vi "Write to Dashboard.vi"   [LabVIEW 2014]
uses:
  Global Variables/Sensor Data (Edited).vi
  <vilib>/Rock Robotics/Network Tables/SD Write Number.vi
  <vilib>/Rock Robotics/Network Tables/SD Write Numeric Array.vi
  <vilib>/Rock Robotics/Network Tables/SD Write Boolean Array.vi
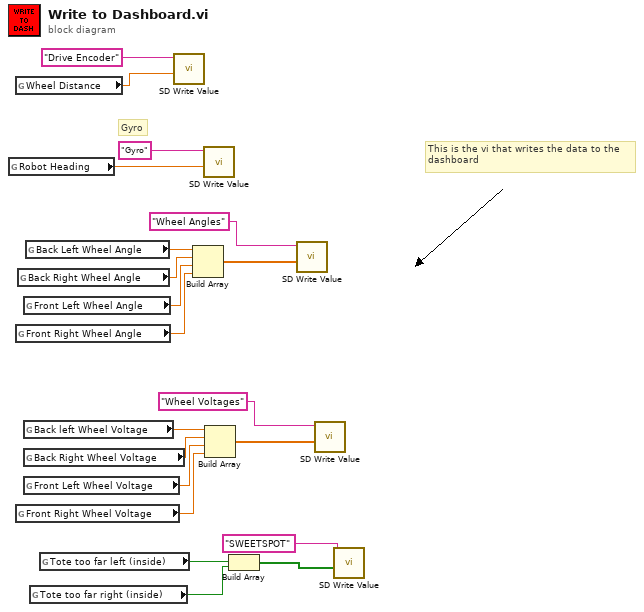
[diagram p0: block diagram]
diagram:
  # "This is the vi that writes the data to the \ndashboard"
  # "Gyro"
  n1 = global read "Sensor Data (Edited).vi" "Robot Heading"() -> (w17:dbl)
  n2 = global read "Sensor Data (Edited).vi" "Wheel Distance"() -> (w19:dbl)
  n3 = global read "Sensor Data (Edited).vi" "Front Right Wheel Angle"() -> (w13:dbl)
  n4 = global read "Sensor Data (Edited).vi" "Front Right Wheel Voltage"() -> (w7:dbl)
  n5 = global read "Sensor Data (Edited).vi" "Back Right Wheel Angle"() -> (w15:dbl)
  n6 = global read "Sensor Data (Edited).vi" "Front Left Wheel Angle"() -> (w14:dbl)
  n7 = global read "Sensor Data (Edited).vi" "Back left Wheel Voltage"() -> (w10:dbl)
  n8 = global read "Sensor Data (Edited).vi" "Back Right Wheel Voltage"() -> (w9:dbl)
  n9 = global read "Sensor Data (Edited).vi" "Front Left Wheel Voltage"() -> (w8:dbl)
  n10 = global read "Sensor Data (Edited).vi" "Back Left Wheel Angle"() -> (w16:dbl)
  n11 = global read "Sensor Data (Edited).vi" "Tote too far right (inside)"() -> (w3:bool)
  n12 = global read "Sensor Data (Edited).vi" "Tote too far left (inside)"() -> (w4:bool)
  n13 = call-poly <vilib>:"SD Write Value.vi"("Numeric"=w19, "Name"="Drive Encoder") -> ()  [unwired: 8 in, 2 out]
  n14 = Build Array(w16, w15, w14, w13) -> (w12:dbl[])
  n15 = call-poly <vilib>:"SD Write Value.vi"("Numeric"=w17, "Name"="Gyro") -> ()  [unwired: 8 in, 2 out]
  n16 = Build Array(w10, w9, w8, w7) -> (w6:dbl[])
  n17 = Build Array(w4, w3) -> (w2:bool[])
  n18 = call-poly <vilib>:"SD Write Value.vi"("Numeric Array"=w12, "Name"="Wheel Angles") -> ()  [unwired: 8 in, 2 out]
  n19 = call-poly <vilib>:"SD Write Value.vi"("Numeric Array"=w6, "Name"="Wheel Voltages") -> ()  [unwired: 8 in, 2 out]
  n20 = call-poly <vilib>:"SD Write Value.vi"("Boolean Array"=w2, "Name"="SWEETSPOT") -> ()  [unwired: 8 in, 2 out]
